vi "extract.vi"   [LabVIEW 2015, in "lv-bin-7zip.lvlib" / "v1.lvlib"]
uses:
  v1.lvlib
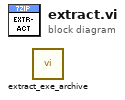
[diagram p0: block diagram]
diagram:
  n1 = call "extract_exe_archive.vi"() -> ()  [unwired: 8 in, 4 out]
